vi "Save_Monitor_Config.vi"   [LabVIEW 2019]
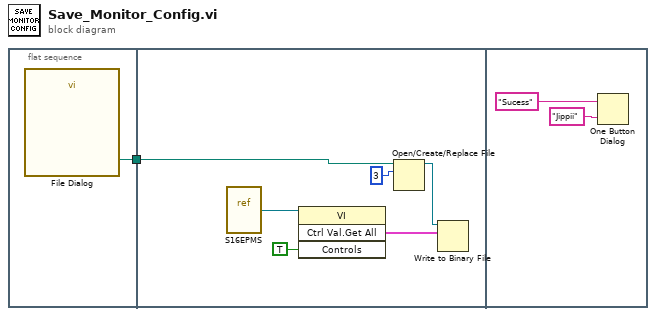
[diagram p0: block diagram]
diagram:
  n1 = flat-sequence {
    tunnel: [w2] -> w1
    tunnel: w1 -> [w3]
    frame #0 {
      n2 = call "File Dialog"() -> ("selected path"=w2:path)  [unwired: 12 in, 3 out]
    }
    frame #1 {
      n3 = vi-ref "S16EPMS.vi"() -> (w7:refnum<vi>)
      n4 = invoke class="VI" method="Ctrl Val.Get All"(reference=w7, "Controls"=TRUE) -> ("Get All Control Values Variant"=w4:cluster{"Name":string, "Variant Data":variant}[])  [unwired: 2 in, 3 out]
      n5 = Open/Create/Replace File(file path (use dialog)=w3, operation (0:open)=3) -> (refnum out=w5:refnum<file>)  [unwired: 4 in, 2 out]
      n6 = Write to Binary File(file (use dialog)=w5, data=w4) -> ()  [unwired: 4 in, 3 out]
    }
    frame #2 {
      n7 = One Button Dialog(message="Sucess", button name ("OK")="Jippii") -> ()  [unwired: 1 out]
    }
  }
